vi "Set Motors Position Setpoint.vi"(8 "error in (no error)":errorcluster, 10 "ccw position (rad)":dbl[](array[numeric])=[0.0, 0.0, 0.0, 0.0, 0.0], 11 "KUKA youBot arm in":refnum<class "NI_Robotics_KUKA youBot Arm.lvclass">) -> (0 "error out":errorcluster, 3 "KUKA youBot arm out":refnum<class "NI_Robotics_KUKA youBot Arm.lvclass">)   [LabVIEW 2017, in "NI_Robotics_KUKA youBot Host.lvlib" / "NI_Robotics_KUKA youBot Arm.lvclass"]
doc: "Sets the position setpoint of the motors attached to the joints of a KUKA youBot arm."
uses:
  <vilib>/robotics/KUKA youBot/Basic Device/Arm/NI_Robotics_KUKA youBot Arm.lvclass
  <vilib>/robotics/KUKA youBot/Basic Device/Arm/NI_Robotics_KUKA youBot Arm.lvclass/NI_Robotics_KUKA youBot Arm.ctl
  <vilib>/robotics/KUKA youBot/Motor/Arm Motor/NI_Robotics_KUKA youBot Arm Motor.lvclass
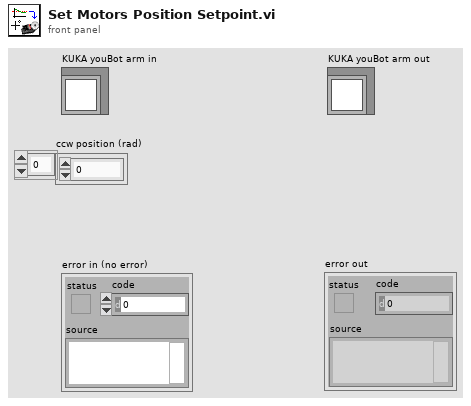
[diagram p1: front panel]
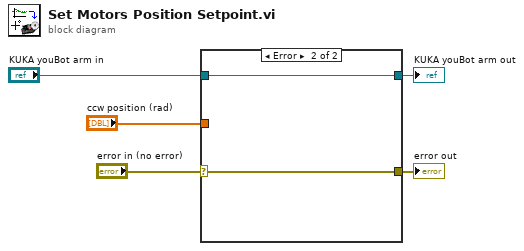
[diagram p0: block diagram]
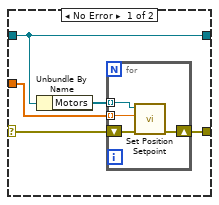
[diagram p2: hidden frame]
diagram:
  n1 = case shown="Error" "error in (no error)" {
    selector: "error in (no error)" -> [w8 w15]
    tunnel: "KUKA youBot arm in" -> [w6 w16]
    tunnel: "ccw position (rad)" -> [w9 _]
    tunnel: [w7 w15] -> w2
    tunnel: [w6 w16] -> w1
    frame No Error {
      n2 = Unbundle By Name(w6) -> ("Motors"=w10:refnum<class "NI_Robotics_KUKA youBot Arm Motor.lvclass">[])
      n3 = for {
        tunnel: w10 -> [w14] mode=indexing
        tunnel: w9 -> [w13] mode=indexing
        shift-right: [w11] -> w7
        shift-left: w8 -> [w12]
        n4 = call-dynamic "Set Position Setpoint.vi"("error in (no error)"=w12, "CCW position (rad)"=w13, "KUKA youBot arm motor in"=w14) -> ("error out"=w11:errorcluster)  [unwired: 7 in, 1 out]
      }
    }
    frame Error {
    }
  }
  "error out" <- w2
  "KUKA youBot arm out" <- w1
